vi "replace notes.vi"(7 "channel type":T2, 8 "error in (no error)":errorcluster, 9 "index of element":i32, 10 "notes":string, 11 "Item Ref in":T1 format="%.0x") -> (0 "error out":errorcluster, 3 "Item Ref out":T1 format="%.0x")   [LabVIEW 2016]
uses:
  <vilib>/NI Veristand/Custom Device API/Custom Device Item Ref.ctl
  FPGA-Addon/Source/System Explorer/SubVIs/Channel Type.ctl
  <vilib>/NI Veristand/Custom Device API/Get Item Property (String Array).vi
  <vilib>/NI Veristand/Custom Device API/Set Item Property (String Array).vi
  <vilib>/NI VeriStand/Custom Device API/Custom Device API.lvlib
  FPGA-Addon/Source/System Explorer/FPGA Addon System Explorer.lvlib
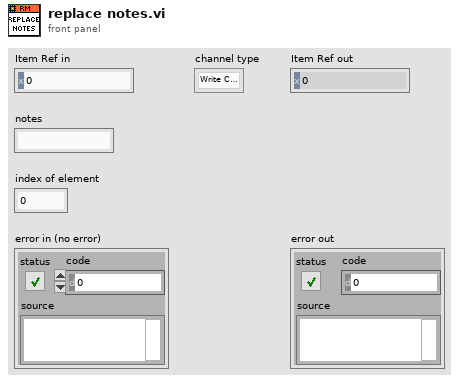
[diagram p1: front panel]
types:
  T1 = typedef "Custom Device API.lvlib/Custom Device Item Ref.ctl" = u64
  T2 = typedef "FPGA Addon System Explorer.lvlib/Channel Type.ctl" = enum16{"Write Channel", "Read Channel", "Write Waveform", "Read Waveform"}
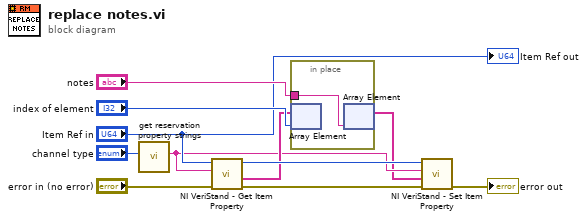
[diagram p0: block diagram]
diagram:
  n1 = call "get reservation property strings.vi"("channel type"="channel type") -> ("reservations"=w2:string)  [unwired: 8 in, 2 out]
  n2 = call-poly <vilib>:"NI VeriStand - Get Item Property.vi"("error in (no error)"="error in (no error)", "Property Name"=w2, "Item Ref in"="Item Ref in") -> ("error out"=w5:errorcluster, "Value"=w7:string[], "Item Ref out"=w11:T1)  [unwired: 5 in, 1 out]
  n3 = in-place {
    in-place-border: "notes" -> [w12]
    n4 = in-place-array #1(w7, "index of element") -> ()  [unwired: 1 out]
    n5 = in-place-array #1(w12) -> (w1:string[])  [unwired: 1 out]
  }
  n6 = call-poly <vilib>:"NI VeriStand - Set Item Property.vi"("error in (no error)"=w5, "Value"=w1, "Property Name"=w2, "Item Ref in"=w11) -> ("error out"=→"error out":errorcluster)  [unwired: 5 in, 2 out]
  "Item Ref out" <- "Item Ref in"
